vi "Parse NT String.vi"(11 "TCP Network Connection in":refnum<k5>) -> (1 "Size":i32=1, 2 "String":string, 3 "TCP Network Connection out":refnum<k5>)   [LabVIEW 2017]
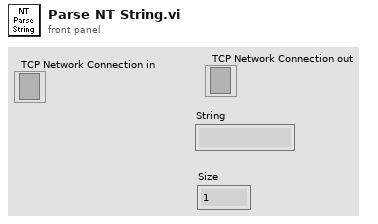
[diagram p1: front panel]
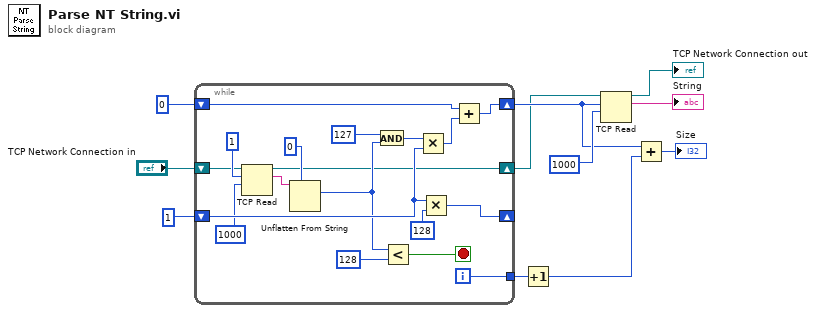
[diagram p0: block diagram]
diagram:
  n1 = while {
    shift-right: [w28] -> w4
    shift-left: u32 0 -> [w29]
    shift-right: [w26] -> _
    shift-left: u32 1 -> [w27]
    tunnel: [w19] -> w8
    shift-right: [w12] -> w1
    shift-left: "TCP Network Connection in" -> [w13]
    i -> [w19]
    stop <- w22 stop-if-true
    n2 = TCP Read(connection ID=w13, bytes to read=1 ("timeout ms (25000)"), 9:1000 ("timeout ms (25000)")) -> (connection ID out=w12:refnum<k5>, data out=w16:string)  [unwired: 2 in, 1 out]
    n3 = Unflatten From String(type=u8 0 ("Size"), binary string=w16) -> (value=w14:u8)  [unwired: 3 in, 2 out]
    n4 = And(x=u8 127, y=w14) -> (x .and. y?=w21:u8)
    n5 = Less?(x=w14, y=u32 128) -> (x < y?=w22:bool)
    n6 = Multiply(x=w21, y=w27) -> (x*y=w24:u32)
    n7 = Multiply(x=w27, y=u32 128) -> (x*y=w26:u32)
    n8 = Add(x=w29, y=w24) -> (x+y=w28:u32)
  }
  n9 = Increment(x=w8) -> (x+1=w3:i32)
  n10 = TCP Read(connection ID=w1, bytes to read=w4, 9:1000 ("timeout ms (25000)")) -> (connection ID out=→"TCP Network Connection out":refnum<k5>, data out=→"String":string)  [unwired: 2 in, 1 out]
  n11 = Add(x=w4, y=w3) -> (x+y=→"Size":u32)
